vi "PrimaryInterfaceGetVariables.vi"(8 "PrimaryInterface":refnum<k24>, 11 "error in":errorcluster) -> (0 "Variables":T1(array[cluster]), 3 "error out":errorcluster)   [LabVIEW 2013, in "UnderAutomation.UniversalRobots.lvlib"]
uses:
  UnderAutomation.UniversalRobots.lvlib
  C:/Users/fg/Documents/UniversalRobots.vi/LabVIEW_2024/UnderAutomation.UniversalRobots/lib/UnderAutomation.UniversalRobots.dll
  LabVIEW_2024/UnderAutomation.UniversalRobots/lib/UnderAutomation.UniversalRobots.dll
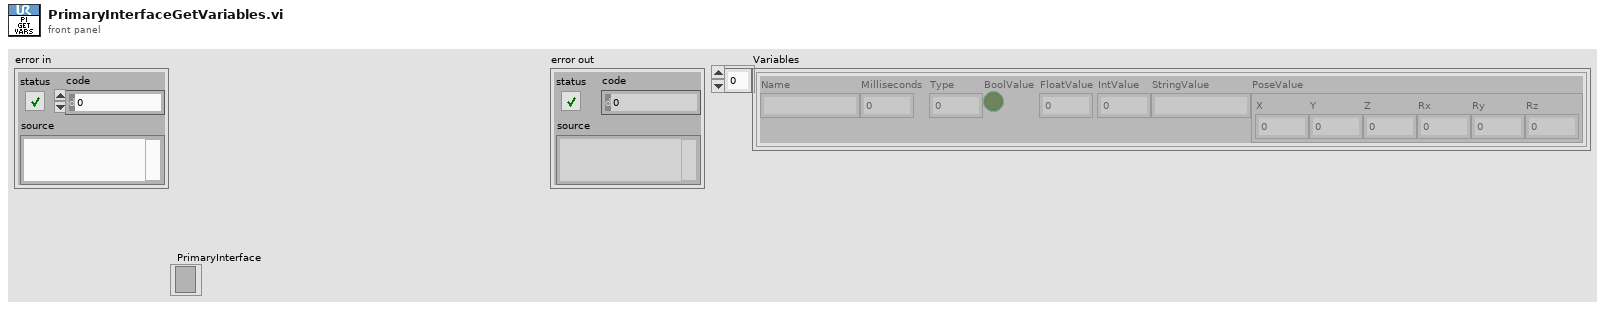
[diagram p1: front panel]
types:
  T1 = cluster{"Name":string, "Milliseconds":i32, "Type":i32, "BoolValue":bool, "FloatValue":sgl, "IntValue":i32, "StringValue":string, "PoseValue":cluster{"X":dbl, "Y":dbl, "Z":dbl, "Rx":dbl, "Ry":dbl, "Rz":dbl}}[]
  T2 = cluster{"Name":string, "Milliseconds":i32, "Type":i32, "BoolValue":bool, "FloatValue":sgl, "IntValue":i32, "StringValue":string, "PoseValue":cluster{"X":dbl, "Y":dbl, "Z":dbl, "Rx":dbl, "Ry":dbl, "Rz":dbl}}
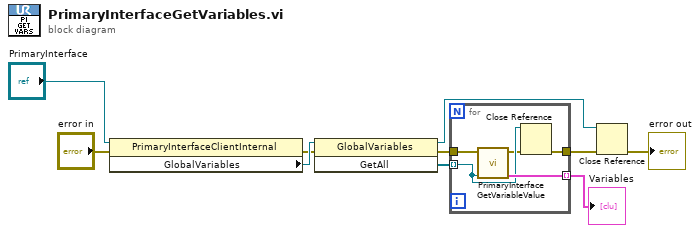
[diagram p0: block diagram]
diagram:
  n1 = property class="PrimaryInterfaceClientInternal"(reference="PrimaryInterface", error in="error in") -> (error out=w5:errorcluster, "GlobalVariables"=w9:refnum<k24>)  [unwired: 1 out]
  n2 = invoke class="GlobalVariables" method="GetAll"(reference=w9, error in=w5) -> (reference out=w1:refnum<k24>, error out=w4:errorcluster, "GetAll"=w8:refnum<k24>[])  [unwired: 1 in]
  n3 = for {
    tunnel: w8 -> [w14] mode=indexing
    tunnel: [w15] -> w7 mode=indexing
    tunnel: w4 -> [w12]
    tunnel: [w11] -> w2
    n4 = call "PrimaryInterfaceGetVariableValue.vi"("Variable"=w14, "error in"=w12) -> ("Value"=w15:T2, "error out"=w13:errorcluster)  [unwired: 8 in]
    n5 = Close Reference(reference=w14, error in (no error)=w13) -> (error out=w11:errorcluster)
  }
  "Variables" <- w7
  n6 = Close Reference(reference=w1, error in (no error)=w2) -> (error out=→"error out":errorcluster)
